vi "Util_Convert I16 to HexString.vi"(4 "Number":i16) -> (1 "HexString":string)   [LabVIEW 2020]
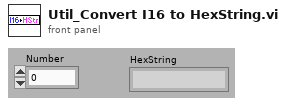
[diagram p1: front panel]
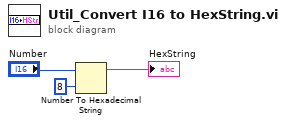
[diagram p0: block diagram]
diagram:
  n1 = Number To Hexadecimal String(1:i16 8 ("width (-)"), 2:"Number") -> (0:→"HexString":string)
